vi "Series Statistical Analysis.vi"() -> ()   [LabVIEW 2023]
doc: "This example shows how to perform statistical analysis on time series using the Statistical Analysis VIs.\n\n<b>Instructions:</b>\n1) Run this VI.\n2) Try and observe different type of statistical analysis."
uses:
  <vilib>/addons/Time Series Analysis/Utilities.llb/TSA Uniform Distribution (Waveform).vi
  <vilib>/addons/Time Series Analysis/Utilities.llb/TSA Normal Distribution (Waveform).vi
  <vilib>/addons/Time Series Analysis/Statistical Analysis.llb/TSA Normal Distribution Test (Waveform).vi
  <vilib>/addons/Time Series Analysis/Statistical Analysis.llb/TSA Mean (Waveform).vi
  <vilib>/addons/Time Series Analysis/Statistical Analysis.llb/TSA Confidence Limits (Waveform).vi
  <vilib>/addons/Time Series Analysis/Statistical Analysis.llb/TSA Deviation and Variance (Waveform).vi
  <vilib>/addons/Time Series Analysis/Statistical Analysis.llb/TSA Skewness and Kurtosis (Waveform).vi
  <vilib>/addons/Time Series Analysis/Statistical Analysis.llb/TSA Entropy (Waveform).vi
  <vilib>/addons/Time Series Analysis/Statistical Analysis.llb/TSA Whiteness Test (Waveform).vi
  <vilib>/addons/Time Series Analysis/Statistical Analysis.llb/TSA Stationarity Test (Waveform).vi
  <vilib>/addons/_Advanced Signal Processing/NI_AdvSigProcTSA.lvlib
panel:
  in  "stop":bool
  in  "Gaussian\nUniform":bool=TRUE
  in  "Confidence level (%)":dbl=95.0
  out "Stationary?":bool
  in  "Confidence level 2 (%)":dbl=99.0
  in  "Confidence level 3 (%)":dbl=95.0
  in  "Weighting":u16(ring) items=["Sample (N-1)", "Population (N)"]
  in  "Confidence level 1 (%)":dbl=95.0
  out "Upper limit of standard deviation":dbl=1.030541966492833 format="%#.4g"
  out "Lower limit of standard deviation":dbl=0.9672699609330174 format="%#.4g"
  in  "Method":u16(ring) items=["Arithmetic", "Geometric", "Trimmed", "Median"]
  out "White?":bool
  out "Lower limit of mean":dbl=-0.02133546920102483 format="%#.4g"
  out "Upper limit of mean":dbl=0.1016165013546939 format="%#.4g"
  out "Shannon entropy":dbl=-758.13588525378
  out "Kurtosis":dbl=2.98978280629767
  out "Skewness":dbl=0.09256293849627177
  out "Standard deviation":dbl=1.002495809316514 format="%#.4g"
  out "Mean":dbl=0.04014051607683453 format="%#.4g"
  in  "Samples":i32=1024
  out "Normal Distribution Test":cluster{"Axis":dbl[], dbl[]}[](graph)
  out "Noise Series":waveform(dbl)(graph)
  # "Overview: Shows how to perform statistical analysis on time series using the Statistical Analysis VIs.\nRequirements: LabVIEW Full Development System, Advanced Signal Processing Toolkit\nInstructions: \n1. Run this VI.\n2. Try and observe different type of statistical analysis.\n3.  Click Stop to stop the VI."
  # "Variance Estimation"
  # "High Order Statistics"
  # "Mean Estimation"
  # "Randomness Test"
  # "Randomness Test"
  # "Entropy"
  # "Stationary Test"
  # "T: Gaussian"
  # "F: Uniform"
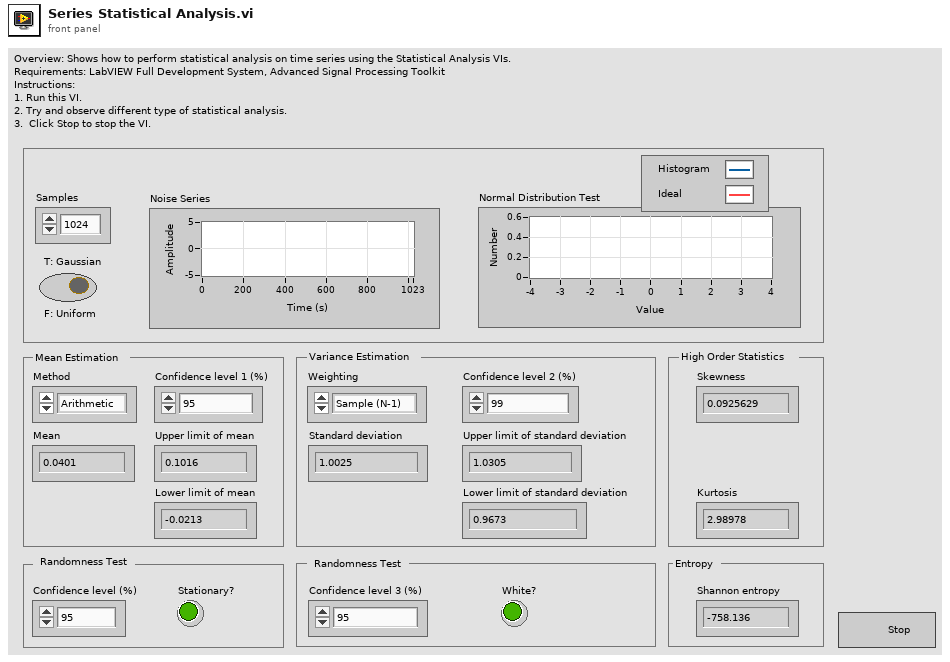
[diagram p1: front panel]
types:
  T1 = enum16{"shannon", "threshold", "sure", "norm", "energy"}
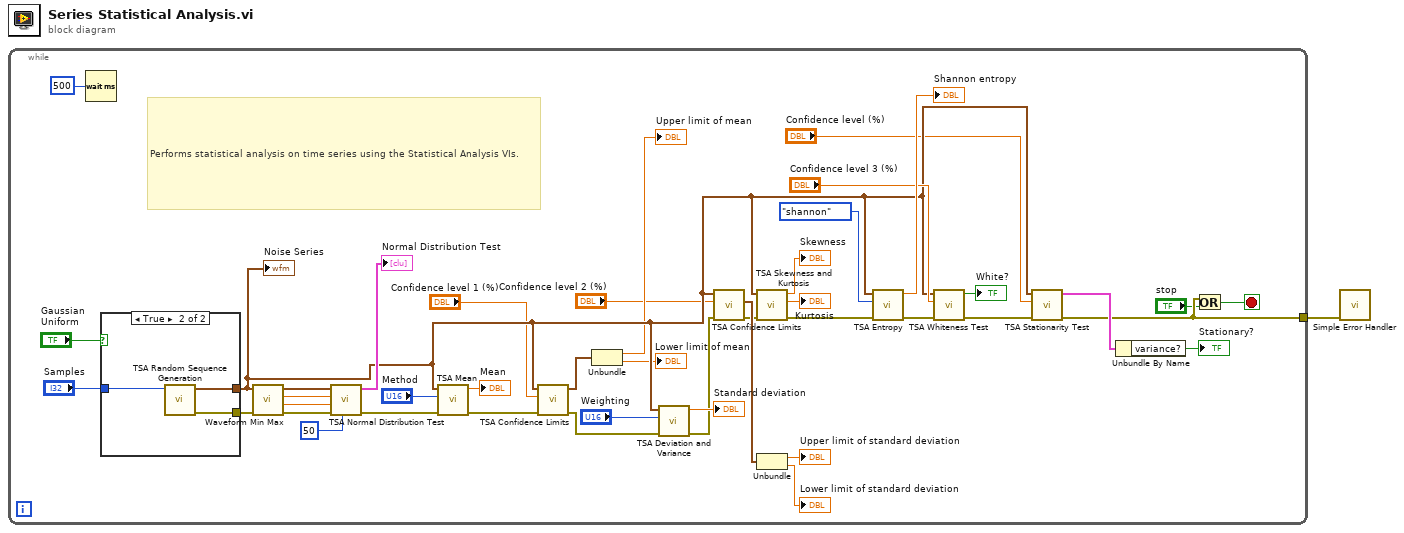
[diagram p0: block diagram]
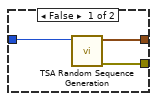
[diagram p2: hidden frame]
diagram:
  n1 = while {
    tunnel: [w4] -> w1
    stop <- w8 stop-if-true
    # "Performs statistical analysis on time series using the Statistical Analysis VIs."
    n2 = Wait (ms)(milliseconds to wait=u32 500 ("millisecond multiple")) -> ()  [unwired: 1 out]
    n3 = case shown="True" "Gaussian\nUniform" {
      tunnel: "Samples" -> [w47 w49]
      tunnel: [w46 w50] -> w28
      tunnel: [w45 w48] -> w6
      frame False {
        n4 = call-poly <vilib>:"TSA Random Sequence Generation.vi"("samples"=w47) -> ("error out"=w45:errorcluster, "Xt"=w46:waveform(dbl))  [unwired: 3 in, 6 out]
      }
      frame True {
        n5 = call-poly <vilib>:"TSA Random Sequence Generation.vi"("samples"=w49) -> ("error out"=w48:errorcluster, "Xt"=w50:waveform(dbl))  [unwired: 3 in, 6 out]
      }
    }
    "Noise Series" <- w28
    n6 = call <vilib>:"Waveform Min Max.vi"("error in (no error)"=w6, "waveform in"=w28) -> ("error out"=w5:errorcluster, "Y min"=w41:dbl, "Y max"=w42:dbl, "waveform out"=w43:waveform(dbl))  [unwired: 6 out]
    n7 = call-poly <vilib>:"TSA Normal Distribution Test.vi"("bins"=50, "error in (no error)"=w5, "min"=w41, "max"=w42, "Xt"=w43) -> ("error out"=w16:errorcluster, "histogram"=→"Normal Distribution Test":cluster{"Axis":dbl[], dbl[]}[])  [unwired: 5 out]
    n8 = call-poly <vilib>:"TSA Mean.vi"("error in (no error)"=w16, "method"="Method", "Xt"=w28) -> ("error out"=w15:errorcluster, "mean"=→"Mean":dbl)  [unwired: 7 out]
    n9 = call-poly <vilib>:"TSA Confidence Limits.vi"("error in (no error)"=w15, "confidence level (%)"="Confidence level 1 (%)", "Xt"=w28) -> ("error out"=w14:errorcluster, "mean limits"=w25:cluster{"upper":dbl, "lower":dbl})  [unwired: 7 out]
    n10 = Unbundle(w25) -> ("upper"=→"Upper limit of mean":dbl, "lower"=→"Lower limit of mean":dbl)
    n11 = call-poly <vilib>:"TSA Deviation and Variance.vi"("error in (no error)"=w14, "weighting"="Weighting", "Xt"=w28) -> ("error out"=w13:errorcluster, "standard deviation"=→"Standard deviation":dbl)  [unwired: 7 out]
    n12 = call-poly <vilib>:"TSA Confidence Limits.vi"("error in (no error)"=w13, "confidence level (%)"="Confidence level 2 (%)", "Xt"=w28) -> ("error out"=w12:errorcluster, "std deviation limits"=w21:cluster{"upper":dbl, "lower":dbl})  [unwired: 7 out]
    n13 = call-poly <vilib>:"TSA Skewness and Kurtosis.vi"("error in (no error)"=w12, "Xt"=w28) -> ("error out"=w11:errorcluster, "kurtosis"=→"Kurtosis":dbl, "skewness"=→"Skewness":dbl)  [unwired: 7 out]
    n14 = Unbundle(w21) -> ("upper"=→"Upper limit of standard deviation":dbl, "lower"=→"Lower limit of standard deviation":dbl)
    n15 = call-poly <vilib>:"TSA Entropy.vi"("error in (no error)"=w11, "method"=T1."shannon" ("mode"), "Xt"=w28) -> ("error out"=w10:errorcluster, "entropy"=→"Shannon entropy":dbl)  [unwired: 7 out]
    n16 = call-poly <vilib>:"TSA Whiteness Test.vi"("error in (no error)"=w10, "confidence level (%)"="Confidence level 3 (%)", "Xt"=w28) -> ("error out"=w9:errorcluster, "white noise?"=→"White?":bool)  [unwired: 7 out]
    n17 = call-poly <vilib>:"TSA Stationarity Test.vi"("error in (no error)"=w9, "confidence level (%)"="Confidence level (%)", "Xt"=w28) -> ("error out"=w4:errorcluster, "stationary"=w19:cluster{"mean?":bool, "variance?":bool})  [unwired: 1 in, 6 out]
    n18 = Unbundle By Name(w19) -> ("variance?"=→"Stationary?":bool)
    n19 = Or(x=w4, y="stop") -> (x .or. y?=w8:bool)
  }
  n20 = call <vilib>:"Simple Error Handler.vi"("error in (no error)"=w1) -> ()  [unwired: 1 in, 8 out]
